vi "cluster_def.vi"() -> ()   [LabVIEW 2016]
uses:
  clusterdef.ctl
panel:
  in  "DeviceConfig":T1
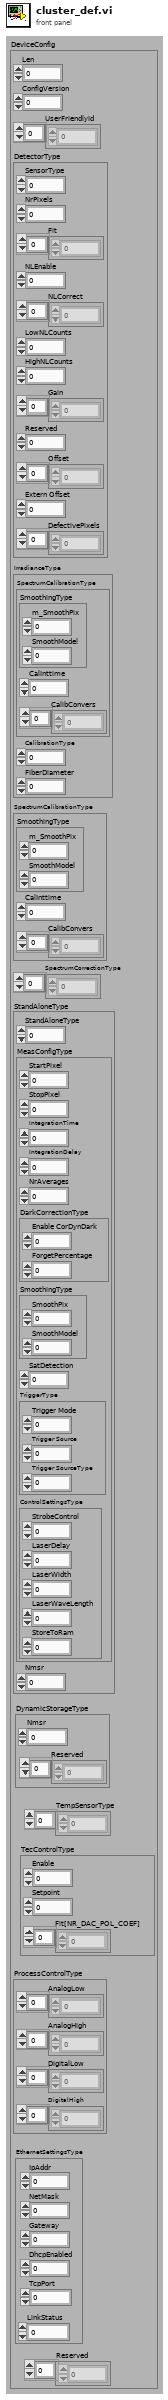
[diagram p1: front panel]
types:
  T1 = typedef "clusterdef.ctl" = cluster{"Len":u16, "ConfigVersion":u16, "UserFriendlyId":u8[], "DetectorType":cluster{"SensorType":u8, "NrPixels":u16, "Fit":sgl[], "NLEnable":u8, "NLCorrect":dbl[], "LowNLCounts":dbl, "HighNLCounts":dbl, "Gain":sgl[], "Reserved":sgl, "Offset":sgl[], "Extern Offset":sgl, "DefectivePixels":u16[]}, "IrradianceType":cluster{"SpectrumCalibrationType":cluster{"SmoothingType":cluster{"m_SmoothPix":u16, "SmoothModel":u8}, "CalInttime":sgl, "CalibConvers":sgl[]}, "CalibrationType":u8, "FiberDiameter":i32}, "SpectrumCalibrationType":cluster{"SmoothingType":cluster{"m_SmoothPix":u16, "SmoothModel":u8}, "CalInttime":sgl, "CalibConvers":sgl[]}, "SpectrumCorrectionType":sgl[], "StandAloneType":cluster{"StandAloneType":u8, "MeasConfigType":cluster{"StartPixel":u16, "StopPixel":u16, "IntegrationTime":sgl, "IntegrationDelay":u32, "NrAverages":u32, "DarkCorrectionType":cluster{"Enable CorDynDark":u8, "ForgetPercentage":u8}, "SmoothingType":cluster{"SmoothPix":u16, "SmoothModel":u8}, "SatDetection":u8, "TriggerType":cluster{"Trigger Mode":u8, "Trigger Source":u8, "Trigger SourceType":u8}, "ControlSettingsType":cluster{"StrobeControl":u16, "LaserDelay":u32, "LaserWidth":u32, "LaserWaveLength":sgl, "StoreToRam":u16}}, "Nmsr":i16}, "DynamicStorageType":cluster{"Nmsr":i32, "Reserved":u8[]}, "TempSensorType":sgl[], "TecControlType":cluster{"Enable":u8, "Setpoint":sgl, "Fit[NR_DAC_POL_COEF]":sgl[]}, "ProcessControlType":cluster{"AnalogLow":sgl[], "AnalogHigh":sgl[], "DigitalLow":sgl[], "DigitalHigh":sgl[]}, "EthernetSettingsType":cluster{"IpAddr":u32, "NetMask":u32, "Gateway":u32, "DhcpEnabled":u8, "TcpPort":u16, "LinkStatus":u8}, "Reserved":u8[]}
  T2 = cluster{"Len":u16, "ConfigVersion":u16, "UserFriendlyId":u8[], "DetectorType":cluster{"SensorType":u8, "NrPixels":u16, "Fit":sgl[], "NLEnable":u8, "NLCorrect":dbl[], "LowNLCounts":dbl, "HighNLCounts":dbl, "Gain":sgl[], "Reserved":sgl, "Offset":sgl[], "Extern Offset":sgl, "DefectivePixels":u16[]}, "IrradianceType":cluster{"SpectrumCalibrationType":cluster{"SmoothingType":cluster{"m_SmoothPix":u16, "SmoothModel":u8}, "CalInttime":sgl, "CalibConvers":sgl[]}, "CalibrationType":u8, "FiberDiameter":i32}, "SpectrumCalibrationType":cluster{"SmoothingType":cluster{"m_SmoothPix":u16, "SmoothModel":u8}, "CalInttime":sgl, "CalibConvers":sgl[]}, "SpectrumCorrectionType":sgl[], "StandAloneType":cluster{"StandAloneType":u8, "MeasConfigType":cluster{"StartPixel":u16, "StopPixel":u16, "IntegrationTime":sgl, "IntegrationDelay":u32, "NrAverages":u32, "DarkCorrectionType":cluster{"Enable CorDynDark":u8, "ForgetPercentage":u8}, "SmoothingType":cluster{"SmoothPix":u16, "SmoothModel":u8}, "SatDetection":u8, "TriggerType":cluster{"Trigger Mode":u8, "Trigger Source":u8, "Trigger SourceType":u8}, "ControlSettingsType":cluster{"StrobeControl":u16, "LaserDelay":u32, "LaserWidth":u32, "LaserWaveLength":sgl, "StoreToRam":u16}}, "Nmsr":i16}, "TempSensorType":sgl[], "TecControlType":cluster{"Enable":u8, "Setpoint":sgl, "Fit[NR_DAC_POL_COEF]":sgl[]}, "ProcessControlType\n":cluster{"AnalogLow":sgl[], "AnalogHigh":sgl[], "DigitalLow":sgl[], "DigitalHigh":sgl[]}, "Reserved":u8[], "DynamicStorageType":cluster{"Nmsr":i32, "Reserved":u8[]}, "EthernetSettingsType":cluster{"IpAddr":u32, "NetMask":u32, "Gateway":u32, "DhcpEnabled":u8, "TcpPort":u16, "LinkStatus":u8}}
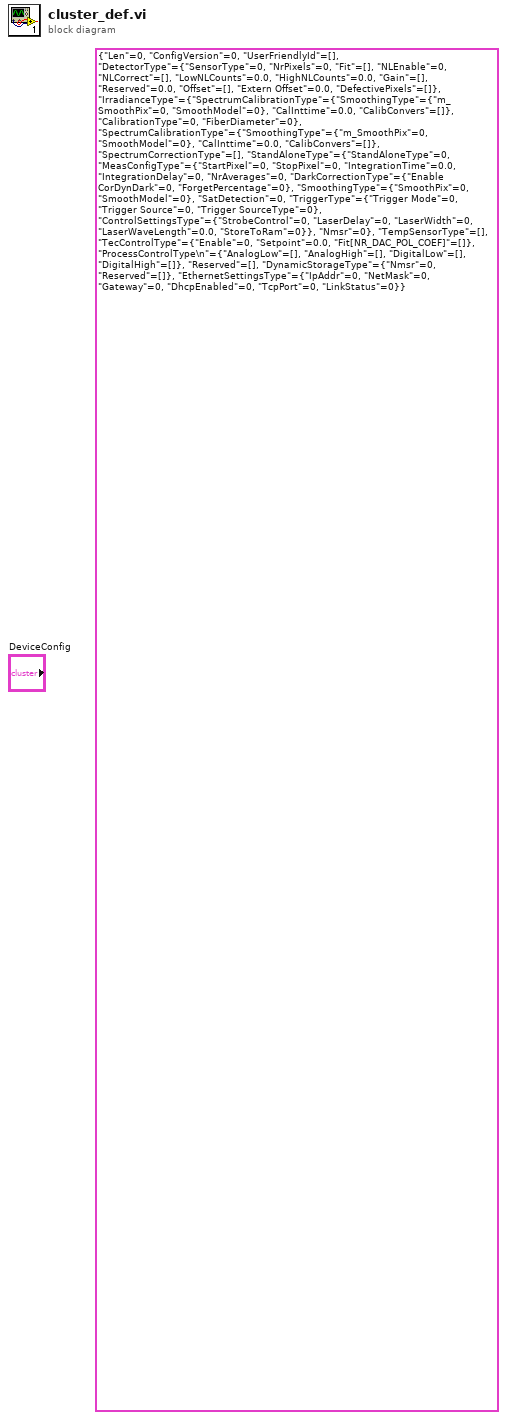
[diagram p0: block diagram]
diagram:
  (unwired) T2 {"Len"=0, "ConfigVersion"=0, "UserFriendlyId"=[], "DetectorType"={"SensorType"=0, "NrPixels"=0, "Fit"=[], "NLEnable"=0, "NLCorrect"=[], "LowNLCounts"=0.0, "HighNLCounts"=0.0, "Gain"=[], "Reserved"=0.0, "Offset"=[], "Extern Offset"=0.0, "DefectivePixels"=[]}, "IrradianceType"={"SpectrumCalibrationType"={"SmoothingType"={"m_SmoothPix"=0, "SmoothModel"=0}, "CalInttime"=0.0, "CalibConvers"=[]}, "CalibrationType"=0, "FiberDiameter"=0}, "SpectrumCalibrationType"={"SmoothingType"={"m_SmoothPix"=0, "SmoothModel"=0}, "CalInttime"=0.0, "CalibConvers"=[]}, "SpectrumCorrectionType"=[], "StandAloneType"={"StandAloneType"=0, "MeasConfigType"={"StartPixel"=0, "StopPixel"=0, "IntegrationTime"=0.0, "IntegrationDelay"=0, "NrAverages"=0, "DarkCorrectionType"={"Enable CorDynDark"=0, "ForgetPercentage"=0}, "SmoothingType"={"SmoothPix"=0, "SmoothModel"=0}, "SatDetection"=0, "TriggerType"={"Trigger Mode"=0, "Trigger Source"=0, "Trigger SourceType"=0}, "ControlSettingsType"={"StrobeControl"=0, "LaserDelay"=0, "LaserWidth"=0, "LaserWaveLength"=0.0, "StoreToRam"=0}}, "Nmsr"=0}, "TempSensorType"=[], "TecControlType"={"Enable"=0, "Setpoint"=0.0, "Fit[NR_DAC_POL_COEF]"=[]}, "ProcessControlType\n"={"AnalogLow"=[], "AnalogHigh"=[], "DigitalLow"=[], "DigitalHigh"=[]}, "Reserved"=[], "DynamicStorageType"={"Nmsr"=0, "Reserved"=[]}, "EthernetSettingsType"={"IpAddr"=0, "NetMask"=0, "Gateway"=0, "DhcpEnabled"=0, "TcpPort"=0, "LinkStatus"=0}} ("DeviceConfig")
